vi "K2400setV.vi"(2 "error in":errorcluster, 3 "Voltage target [V]":dbl, 4 "VISA Resource Name":refnum<visa-resource-name>="GPIB0::11::INSTR") -> (0 "error out":errorcluster, 1 "VISA resource name out":refnum<visa-resource-name>)   [LabVIEW 2011]
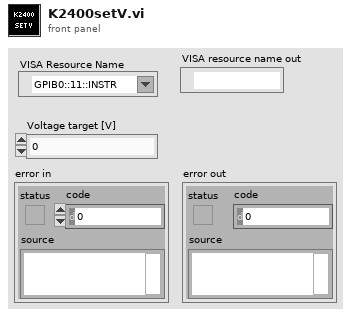
[diagram p1: front panel]
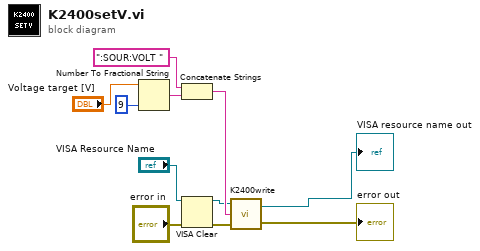
[diagram p0: block diagram]
diagram:
  n1 = Number To Fractional String(number="Voltage target [V]", precision (6)=9) -> (F-format string=w11:string)  [unwired: 2 out]
  n2 = Concatenate Strings(":SOUR:VOLT ", w11) -> (w8:string)
  n3 = VISA Clear(VISA resource name="VISA Resource Name", error in (no error)="error in") -> (VISA resource name out=w3:refnum<visa-resource-name>, error out=w5:errorcluster)
  n4 = call "K2400write.vi"("error in (no error)"=w5, "Command"=w8, "VISA Resource Name"=w3) -> ("error out"=→"error out":errorcluster, "VISA resource name out"=→"VISA resource name out":refnum<visa-resource-name>)
